vi "JSON to LVJSON.vi"(8 "error in (no error)":errorcluster, 11 "JSON in":string) -> (0 "error out":errorcluster, 3 "Root Element out":T1)   [LabVIEW 2019, in "labview_json.lvlib"]
uses:
  labview_json.lvlib
  Element.ctl
  Element Type.ctl
  <vilib>/Utility/error.llb/Error Cluster From Error Code.vi
  <vilib>/ErrorRing/Error Ring.xnode
  <vilib>/regexp/Match Regular Expression.xnode
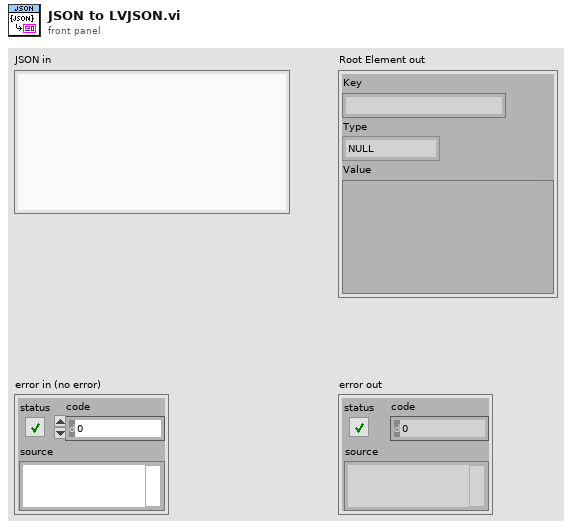
[diagram p1: front panel]
types:
  T1 = typedef "labview_json.lvlib/Element.ctl" = cluster{"Key":string, "Type":T2, "Value":variant}
  T2 = typedef "labview_json.lvlib/Element Type.ctl" = enum8{"NULL", "OBJECT", "ARRAY", "BOOL", "INT", "UINT", "FLOAT", "STRING"}
  T3 = cluster{"Kind":enum8{"Root", "Object", "Array"}, "Name":string, "Values":T1[]}[]
  T4 = cluster{"Kind":enum8{"Root", "Object", "Array"}, "Name":string, "Values":T1[]}
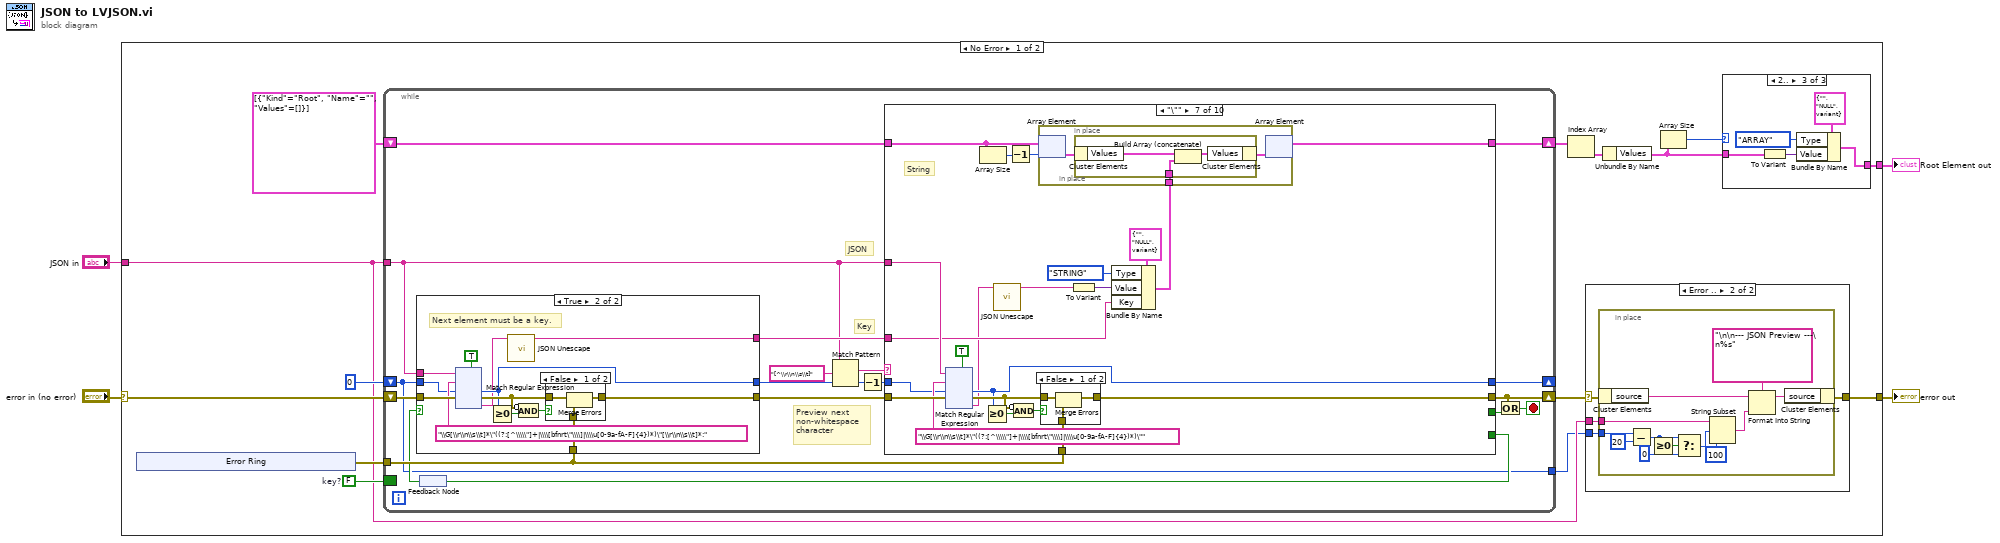
[diagram p0: block diagram]
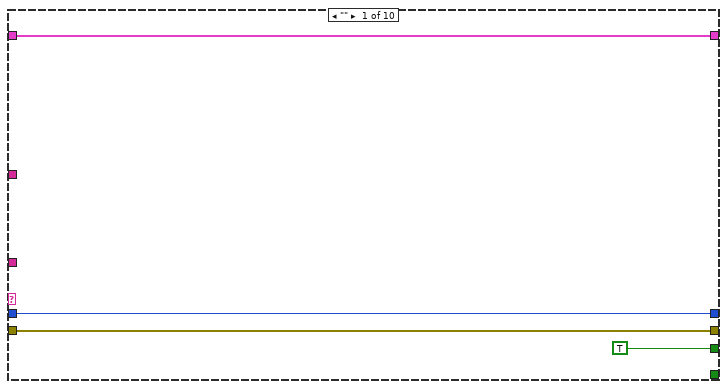
[diagram p5: hidden frame]
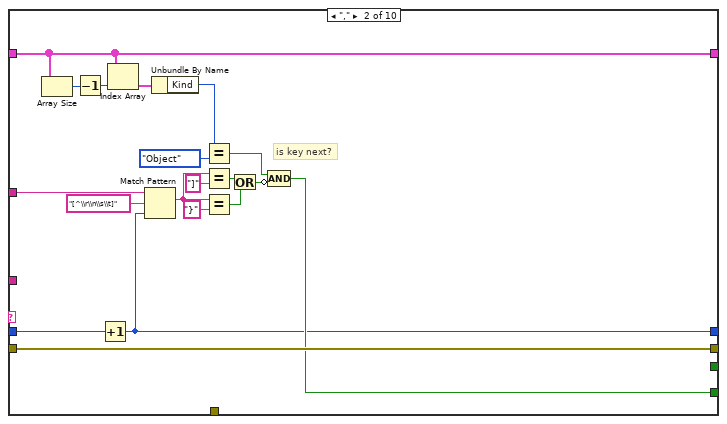
[diagram p6: hidden frame]
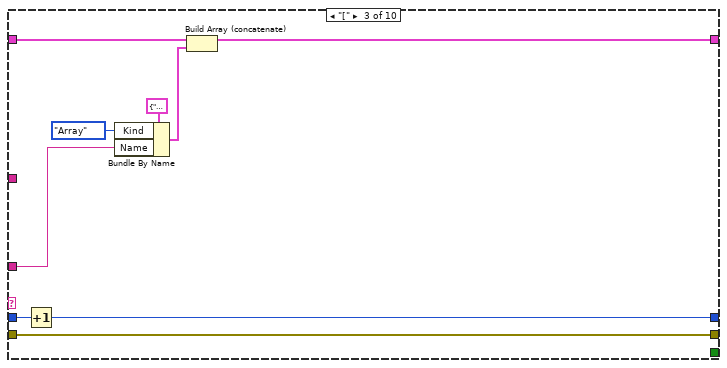
[diagram p7: hidden frame]
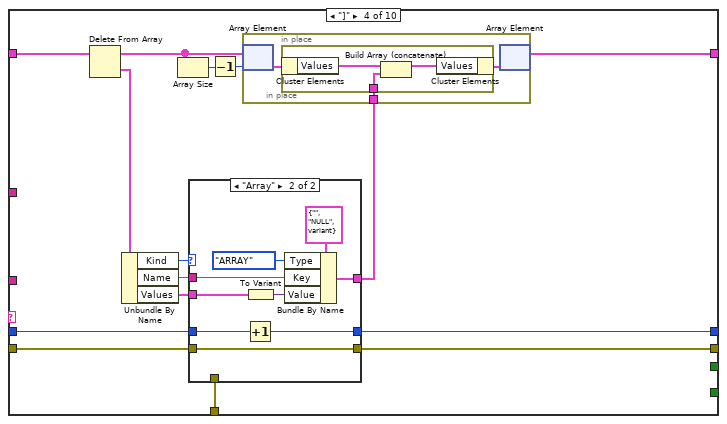
[diagram p8: hidden frame]
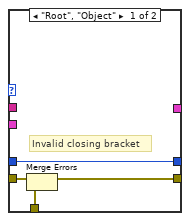
[diagram p9: hidden frame]
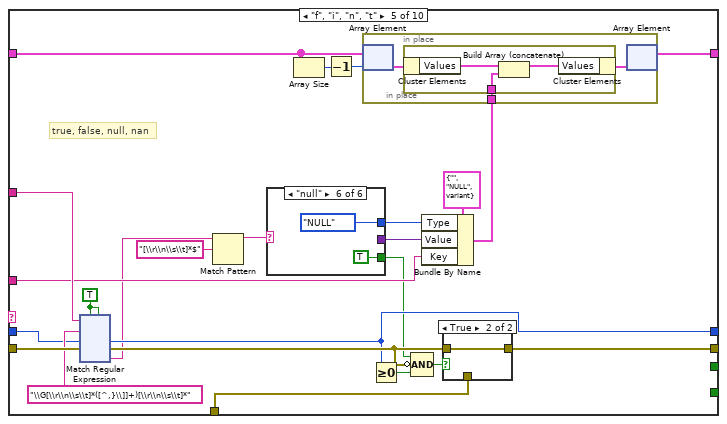
[diagram p10: hidden frame]
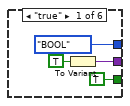
[diagram p11: hidden frame]
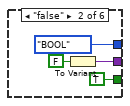
[diagram p12: hidden frame]
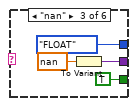
[diagram p13: hidden frame]
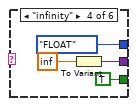
[diagram p14: hidden frame]
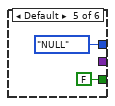
[diagram p15: hidden frame]
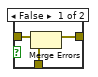
[diagram p16: hidden frame]
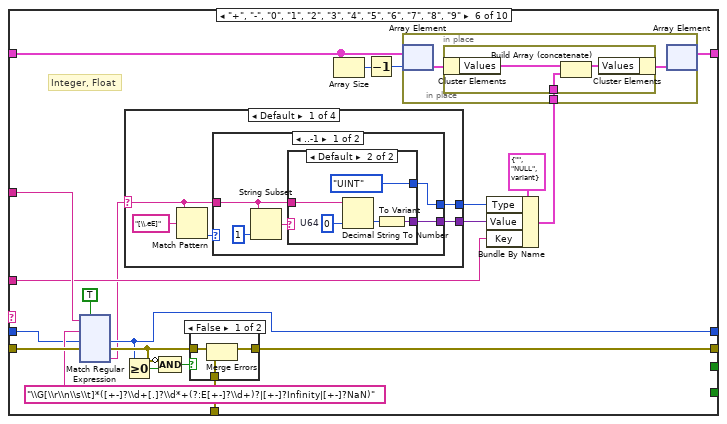
[diagram p17: hidden frame]
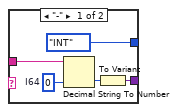
[diagram p18: hidden frame]
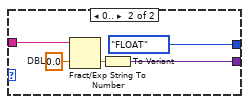
[diagram p19: hidden frame]
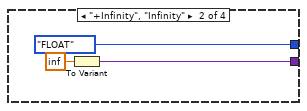
[diagram p20: hidden frame]
diagram:
  n1 = case shown="No Error" "error in (no error)" {
    selector: "error in (no error)" -> [w14 w819]
    tunnel: [w9 _] -> w3
    tunnel: [w8 w819] -> w2
    tunnel: "JSON in" -> [w6 _]
    frame No Error {
      w15 = FALSE  # key?
      n2 = xnode "Error Ring"() -> ("error out"=w13:errorcluster)
      n3 = while {
        tunnel: w6 -> [w48]
        shift-right: [w58] -> w16
        shift-left: T3 [{"Kind"=enum."Root", "Name"="", "Values"=[]}] ("Context") -> [w57]
        shift-right: [w56] -> _
        shift-left: 0 ("Offset in (0)") -> [w40]
        border: w15 -> [_]
        shift-right: [w44] -> w7
        shift-left: w14 -> [w55]
        tunnel: w13 -> [w47]
        tunnel: [w40] -> w5
        stop <- w43 stop-if-true
        # "JSON"
        # "Key"
        # "Preview next\nnon-whitespace\ncharacter"
        n4 = feedback #1() -> (w46:bool)
        n5 = case shown="True" w46 {
          tunnel: w48 -> [_ w72]
          tunnel: w55 -> [w60 w71]
          tunnel: w40 -> [w59 w69]
          tunnel: [w60 w64] -> w51
          tunnel: w47 -> [_ w66]
          tunnel: [w59 w63] -> w53
          tunnel: [_ w61] -> w50
          frame False {
            # "No key"
            # "Next element can be anything"
          }
          frame True {
            # "Next element must be a key."
            n6 = xnode "Match Regular Expression"("input string"=w72, "regular expression"="\\G[\\r\\n\\s\\t]*\"((?:[^\\\\\"]+|\\\\[bfnrt\"\\\\]|\\\\u[0-9a-fA-F]{4})*)\"[\\r\\n\\s\\t]*:", "offset (0)"=w69, "error in"=w71, "multiline? (F)"=TRUE) -> ("offset past match"=w63:i32, "error out"=w65:errorcluster, "submatch 1"=w62:string)  [unwired: 1 in, 3 out]
            n7 = Greater Or Equal To 0?(x=w63) -> (x >= 0?=w68:bool)
            n8 = call "JSON Unescape.vi"("Escaped String"=w62) -> ("String out"=w61:string)  [unwired: 9 in, 1 out]
            n9 = Compound Arithmetic op=AND(invert w65, w68) -> (w67:bool)
            n10 = case shown="False" w67 {
              tunnel: w66 -> [w74 _]
              tunnel: w65 -> [w76 w77]
              tunnel: [w75 w77] -> w64
              frame False {
                n11 = Merge Errors(w76, w74) -> (w75:errorcluster)
              }
              frame True {
              }
            }
          }
        }
        n12 = Match Pattern(string=w48, regular expression="[^\\r\\n\\s\\t]", offset (0)=w53) -> (match substring=w52:string, offset past match=w49:i32)  [unwired: 2 out]
        n13 = Decrement(x=w49) -> (x-1=w45:i32)
        n14 = case shown="\"\\\"\"" w52 {
          tunnel: [TRUE _ _ _ _ _ _ _ _ _] -> w42
          tunnel: w48 -> [_ w202 _ _ w276 w443 w626 w764 _ _]
          tunnel: w45 -> [w195 w201 w220 w228 w265 w432 w617 w767 w775 w809]
          tunnel: [w196 w216 w224 w235 w281 w448 w630 w771 w782 w811] -> w58
          tunnel: w57 -> [w196 w216 w225 w240 w280 w447 w629 w772 w787 w811]
          tunnel: [w195 w198 w218 w229 w269 w436 w620 w760 w776 w809] -> w56
          tunnel: [w194 w200 w219 w232 w267 w434 w619 w766 w779 w808] -> w44
          tunnel: w51 -> [w194 w200 w219 w231 w277 w444 w627 w766 w778 w810]
          tunnel: w50 -> [_ _ w222 _ w264 w431 w616 w769 _ _]
          tunnel: w47 -> [_ _ _ w230 w270 w437 w621 _ w777 w807]
          tunnel: [_ w199 _ _ _ _ _ w761 _ _] -> w41
          frame "" {
          }
          frame "," {
            # "is key next?"
            n15 = Array Size(array=w216) -> (size(s)=w215:i32)
            n16 = Decrement(x=w215) -> (x-1=w214:i32)
            n17 = Increment(x=w201) -> (x+1=w198:i32)
            n18 = Index Array(array=w216, index=w214) -> (element=w213:T4)
            n19 = Match Pattern(string=w202, regular expression="[^\\r\\n\\s\\t]", offset (0)=w198) -> (match substring=w205:string)  [unwired: 3 out]
            n20 = Unbundle By Name(w213) -> ("Kind"=w204:enum8{"Root", "Object", "Array"})
            n21 = Equal?(x=w204, y=enum8{"Root", "Object", "Array"}."Object") -> (x = y?=w208:bool)
            n22 = Equal?(x=w205, y="]") -> (x = y?=w210:bool)
            n23 = Equal?(x=w205, y="}") -> (x = y?=w209:bool)
            n24 = Or(x=w210, y=w209) -> (x .or. y?=w207:bool)
            n25 = Compound Arithmetic op=AND(w208, invert w207) -> (w199:bool)
          }
          frame "[" {
            n26 = Increment(x=w220) -> (x+1=w218:i32)
            n27 = Bundle By Name(cluster=T4 {"Kind"=enum."Root", "Name"="", "Values"=[]} ("Context"), "Kind"=enum8{"Root", "Object", "Array"}."Array", "Name"=w222) -> (w223:T4)
            n28 = Build Array (concatenate)(w225, w223) -> (w224:T3)
          }
          frame "]" {
            n29 = Delete From Array(array=w240) -> (deleted portion=w239:T4, array with subset deleted=w236:T3)  [unwired: 2 in]
            n30 = Unbundle By Name(w239) -> ("Kind"=w234:enum8{"Root", "Object", "Array"}, "Name"=w227:string, "Values"=w233:T1[])
            n31 = Array Size(array=w236) -> (size(s)=w238:i32)
            n32 = case shown="\"Array\"" w234 {
              tunnel: w233 -> [_ w246]
              tunnel: [w243 w252] -> w232
              tunnel: w231 -> [w244 w252]
              tunnel: w230 -> [w242 _]
              tunnel: [w241 w251] -> w229
              tunnel: w228 -> [w241 w253]
              tunnel: [_ w247] -> w226
              tunnel: w227 -> [_ w245]
              frame "Root", "Object" {
                # "Invalid closing bracket"
                n33 = Merge Errors(w244, w242) -> (w243:errorcluster)
              }
              frame "Array" {
                n34 = Increment(x=w253) -> (x+1=w251:i32)
                n35 = To Variant(anything=w246) -> (Variant=w249:variant)
                n36 = Bundle By Name(cluster=T1 {"Key"="", "Type"=enum."NULL", "Value"=variant} ("Value"), "Type"=Element_Type."ARRAY", "Key"=w245, "Value"=w249) -> (w247:T1)
              }
            }
            n37 = Decrement(x=w238) -> (x-1=w237:i32)
            n38 = in-place {
              in-place-border: w226 -> [w255]
              n39 = in-place-array #2(w236, w237) -> (w256:T4)
              n40 = in-place {
                in-place-border: w255 -> [w257]
                n41 = in-place-cluster #3(w256) -> ("Values"=w259:T1[])
                n42 = Build Array (concatenate)(w259, w257) -> (w258:T1[])
                n43 = in-place-cluster #3("Values"=w258) -> (w254:T4)
              }
              n44 = in-place-array #2(w254) -> (w235:T3)  [unwired: 1 out]
            }
          }
          frame "f", "i", "n", "t" {
            w274 = TRUE ("ignore case? (F)")
            # "true, false, null, nan"
            n45 = xnode "Match Regular Expression"("input string"=w276, "regular expression"="\\G[\\r\\n\\s\\t]*([^,}\\]]+)[\\r\\n\\s\\t]*", "offset (0)"=w265, "error in"=w277, "ignore case? (F)"=w274, "multiline? (F)"=w274) -> ("offset past match"=w269:i32, "error out"=w271:errorcluster, "submatch 1"=w261:string)  [unwired: 3 out]
            n46 = Match Pattern(string=w261, regular expression="[\\r\\n\\s\\t]*$") -> (before substring=w260:string)  [unwired: 1 in, 3 out]
            n47 = case shown="\"null\"" w260 {
              tunnel: [Element_Type."BOOL" ("Type") Element_Type."BOOL" ("Type") Element_Type."FLOAT" ("Type") Element_Type."FLOAT" ("Type") Element_Type."NULL" ("Type") Element_Type."NULL" ("Type")] -> w278
              tunnel: [w285 w289 w294 w298 _ _] -> w268
              tunnel: [TRUE TRUE TRUE TRUE FALSE TRUE] -> w263
              frame "true" {
                n48 = To Variant(anything=TRUE) -> (Variant=w285:variant)
              }
              frame "false" {
                n49 = To Variant(anything=FALSE) -> (Variant=w289:variant)
              }
              frame "nan" {
                n50 = To Variant(anything=nan) -> (Variant=w294:variant)
              }
              frame "infinity" {
                n51 = To Variant(anything=inf) -> (Variant=w298:variant)
              }
              frame Default {
              }
              frame "null" {
              }
            }
            n52 = Array Size(array=w280) -> (size(s)=w283:i32)
            n53 = Decrement(x=w283) -> (x-1=w282:i32)
            n54 = Greater Or Equal To 0?(x=w269) -> (x >= 0?=w272:bool)
            n55 = Compound Arithmetic op=AND(w263, invert w271, w272) -> (w273:bool)
            n56 = Bundle By Name(cluster=T1 {"Key"="", "Type"=enum."NULL", "Value"=variant} ("Value"), "Type"=w278, "Value"=w268, "Key"=w264) -> (w266:T1)
            n57 = in-place {
              in-place-border: w266 -> [w425]
              n58 = in-place-array #4(w280, w282) -> (w426:T4)
              n59 = in-place {
                in-place-border: w425 -> [w427]
                n60 = in-place-cluster #5(w426) -> ("Values"=w429:T1[])
                n61 = Build Array (concatenate)(w429, w427) -> (w428:T1[])
                n62 = in-place-cluster #5("Values"=w428) -> (w424:T4)
              }
              n63 = in-place-array #4(w424) -> (w281:T3)  [unwired: 1 out]
            }
            n64 = case shown="True" w273 {
              tunnel: w270 -> [w304 _]
              tunnel: w271 -> [w306 w307]
              tunnel: [w305 w307] -> w267
              frame False {
                n65 = Merge Errors(w306, w304) -> (w305:errorcluster)
              }
              frame True {
              }
            }
          }
          frame "+", "-", "0", "1", "2", "3", "4", "5", "6", "7", "8", "9" {
            # "Integer, Float"
            n66 = xnode "Match Regular Expression"("input string"=w443, "regular expression"="\\G[\\r\\n\\s\\t]*([+-]?\\d+[.]?\\d*+(?:E[+-]?\\d+)?|[+-]?Infinity|[+-]?NaN)", "offset (0)"=w432, "error in"=w444, "ignore case? (F)"=TRUE) -> ("offset past match"=w436:i32, "error out"=w438:errorcluster, "submatch 1"=w430:string)  [unwired: 1 in, 3 out]
            n67 = Greater Or Equal To 0?(x=w436) -> (x >= 0?=w439:bool)
            n68 = case shown="Default" w430 {
              selector: w430 -> [w453 _ _ _]
              tunnel: [w451 Element_Type."FLOAT" ("Type") Element_Type."FLOAT" ("Type") Element_Type."FLOAT" ("Type")] -> w445
              tunnel: [w452 w477 w480 w483] -> w435
              frame Default {
                n69 = Match Pattern(string=w453, regular expression="[\\.eE]") -> (offset past match=w455:i32)  [unwired: 1 in, 3 out]
                n70 = case shown="..-1" w455 {
                  tunnel: w453 -> [w459 w475]
                  tunnel: [w458 w472] -> w452
                  tunnel: [w456 Element_Type."FLOAT" ("Type")] -> w451
                  frame ..-1 {
                    n71 = String Subset(string=w459, length (rest)=1 ("length (rest)")) -> (substring=w457:string)  [unwired: 1 in]
                    n72 = case shown="Default" w457 {
                      tunnel: w459 -> [w465 w470]
                      tunnel: [w462 w467] -> w458
                      tunnel: [Element_Type."INT" ("Type") Element_Type."UINT" ("Type")] -> w456
                      frame "-" {
                        w464 = i64 0  # I64
                        n73 = Decimal String To Number(string=w465, default (0L)=w464) -> (number=w463:i64)  [unwired: 1 in, 1 out]
                        n74 = To Variant(anything=w463) -> (Variant=w462:variant)
                      }
                      frame Default {
                        w469 = u64 0  # U64
                        n75 = Decimal String To Number(string=w470, default (0L)=w469) -> (number=w468:u64)  [unwired: 1 in, 1 out]
                        n76 = To Variant(anything=w468) -> (Variant=w467:variant)
                      }
                    }
                  }
                  frame 0.. {
                    w474 = 0.0  # DBL
                    n77 = Fract/Exp String To Number(string=w475, default (0 dbl)=w474) -> (number=w473:dbl)  [unwired: 2 in, 1 out]
                    n78 = To Variant(anything=w473) -> (Variant=w472:variant)
                  }
                }
              }
              frame "+Infinity", "Infinity" {
                n79 = To Variant(anything=inf) -> (Variant=w477:variant)
              }
              frame "-Infinity" {
                n80 = To Variant(anything=-inf) -> (Variant=w480:variant)
              }
              frame "+NaN", "-NaN", "NaN" {
                n81 = To Variant(anything=nan) -> (Variant=w483:variant)
              }
            }
            n82 = Compound Arithmetic op=AND(invert w438, w439) -> (w440:bool)
            n83 = case shown="False" w440 {
              tunnel: w437 -> [w485 _]
              tunnel: w438 -> [w487 w488]
              tunnel: [w486 w488] -> w434
              frame False {
                n84 = Merge Errors(w487, w485) -> (w486:errorcluster)
              }
              frame True {
              }
            }
            n85 = Array Size(array=w447) -> (size(s)=w450:i32)
            n86 = Decrement(x=w450) -> (x-1=w449:i32)
            n87 = Bundle By Name(cluster=T1 {"Key"="", "Type"=enum."NULL", "Value"=variant} ("Value"), "Type"=w445, "Value"=w435, "Key"=w431) -> (w433:T1)
            n88 = in-place {
              in-place-border: w433 -> [w606]
              n89 = in-place-array #6(w447, w449) -> (w607:T4)
              n90 = in-place {
                in-place-border: w606 -> [w608]
                n91 = in-place-cluster #7(w607) -> ("Values"=w610:T1[])
                n92 = Build Array (concatenate)(w610, w608) -> (w609:T1[])
                n93 = in-place-cluster #7("Values"=w609) -> (w605:T4)
              }
              n94 = in-place-array #6(w605) -> (w448:T3)  [unwired: 1 out]
            }
          }
          frame "\"" {
            # "String"
            n95 = xnode "Match Regular Expression"("input string"=w626, "regular expression"="\\G[\\r\\n\\s\\t]*\"((?:[^\\\\\"]+|\\\\[bfnrt\"\\\\]|\\\\u[0-9a-fA-F]{4})*)\"", "offset (0)"=w617, "error in"=w627, "multiline? (F)"=TRUE ("ignore case? (F)")) -> ("offset past match"=w620:i32, "error out"=w622:errorcluster, "submatch 1"=w613:string)  [unwired: 1 in, 3 out]
            n96 = Array Size(array=w629) -> (size(s)=w632:i32)
            n97 = Greater Or Equal To 0?(x=w620) -> (x >= 0?=w623:bool)
            n98 = call "JSON Unescape.vi"("Escaped String"=w613) -> ("String out"=w612:string)  [unwired: 9 in, 1 out]
            n99 = Decrement(x=w632) -> (x-1=w631:i32)
            n100 = Compound Arithmetic op=AND(invert w622, w623) -> (w624:bool)
            n101 = case shown="False" w624 {
              tunnel: w621 -> [w633 _]
              tunnel: w622 -> [w635 w636]
              tunnel: [w634 w636] -> w619
              frame False {
                n102 = Merge Errors(w635, w633) -> (w634:errorcluster)
              }
              frame True {
              }
            }
            n103 = To Variant(anything=w612) -> (Variant=w611:variant)
            n104 = Bundle By Name(cluster=T1 {"Key"="", "Type"=enum."NULL", "Value"=variant} ("Value"), "Type"=Element_Type."STRING", "Value"=w611, "Key"=w616) -> (w618:T1)
            n105 = in-place {
              in-place-border: w618 -> [w754]
              n106 = in-place-array #8(w629, w631) -> (w755:T4)
              n107 = in-place {
                in-place-border: w754 -> [w756]
                n108 = in-place-cluster #9(w755) -> ("Values"=w758:T1[])
                n109 = Build Array (concatenate)(w758, w756) -> (w757:T1[])
                n110 = in-place-cluster #9("Values"=w757) -> (w753:T4)
              }
              n111 = in-place-array #8(w753) -> (w630:T3)  [unwired: 1 out]
            }
          }
          frame "{" {
            # "Is key next?"
            n112 = Increment(x=w767) -> (x+1=w760:i32)
            n113 = Bundle By Name(cluster=T4 {"Kind"=enum."Root", "Name"="", "Values"=[]} ("Context"), "Kind"=enum8{"Root", "Object", "Array"}."Object", "Name"=w769) -> (w770:T4)
            n114 = Match Pattern(string=w764, regular expression="[^\\r\\n\\s\\t]", offset (0)=w760) -> (match substring=w763:string)  [unwired: 3 out]
            n115 = Build Array (concatenate)(w772, w770) -> (w771:T3)
            n116 = Not Equal?(x=w763, y="}") -> (x != y?=w761:bool)
          }
          frame "}" {
            n117 = Delete From Array(array=w787) -> (deleted portion=w786:T4, array with subset deleted=w783:T3)  [unwired: 2 in]
            n118 = Unbundle By Name(w786) -> ("Kind"=w781:enum8{"Root", "Object", "Array"}, "Name"=w774:string, "Values"=w780:T1[])
            n119 = Array Size(array=w783) -> (size(s)=w785:i32)
            n120 = case shown="\"Object\"" w781 {
              tunnel: w780 -> [_ w793]
              tunnel: [w790 w799] -> w779
              tunnel: w778 -> [w791 w799]
              tunnel: w777 -> [w789 _]
              tunnel: [w788 w798] -> w776
              tunnel: w775 -> [w788 w800]
              tunnel: [_ w794] -> w773
              tunnel: w774 -> [_ w792]
              frame "Root", "Array" {
                # "Invalid closing bracket"
                n121 = Merge Errors(w791, w789) -> (w790:errorcluster)
              }
              frame "Object" {
                n122 = Increment(x=w800) -> (x+1=w798:i32)
                n123 = To Variant(anything=w793) -> (Variant=w796:variant)
                n124 = Bundle By Name(cluster=T1 {"Key"="", "Type"=enum."NULL", "Value"=variant} ("Value"), "Type"=Element_Type."OBJECT", "Key"=w792, "Value"=w796) -> (w794:T1)
              }
            }
            n125 = Decrement(x=w785) -> (x-1=w784:i32)
            n126 = in-place {
              in-place-border: w773 -> [w802]
              n127 = in-place-array #10(w783, w784) -> (w803:T4)
              n128 = in-place {
                in-place-border: w802 -> [w804]
                n129 = in-place-cluster #11(w803) -> ("Values"=w806:T1[])
                n130 = Build Array (concatenate)(w806, w804) -> (w805:T1[])
                n131 = in-place-cluster #11("Values"=w805) -> (w801:T4)
              }
              n132 = in-place-array #10(w801) -> (w782:T3)  [unwired: 1 out]
            }
          }
          frame Default {
            # "Invalid value"
            n133 = Merge Errors(w810, w807) -> (w808:errorcluster)
          }
        }
        n134 = feedback-in #1(w41) -> ()
        n135 = Or(x=w44, y=w42) -> (x .or. y?=w43:bool)
      }
      n136 = Index Array(array=w16) -> (element=w11:T4)  [unwired: 1 in]
      n137 = case shown="Error .." w7 {
        selector: w7 -> [w19 w23]
        tunnel: [w19 w20] -> w8
        tunnel: w6 -> [_ w22]
        tunnel: w5 -> [_ w21]
        frame No Error {
        }
        frame Error {
          n138 = in-place {
            in-place-border: w22 -> [w35]
            in-place-border: w21 -> [w24]
            n139 = in-place-cluster #12(w23) -> ("source"=w32:string)
            n140 = Subtract(x=w24, y=20 ("x")) -> (x-y=w28:i32)
            n141 = Greater Or Equal To 0?(x=w28) -> (x >= 0?=w29:bool)
            n142 = Select(t=w28, s=w29, f=0) -> (s? t:f=w26:i32)
            n143 = String Subset(string=w35, offset (0)=w26, length (rest)=100 ("length (rest)")) -> (substring=w25:string)
            n144 = Format Into String(format string="\n\n--- JSON Preview ---\n%s", initial string=w32, w25) -> (resulting string=w31:string)  [unwired: 1 in, 1 out]
            n145 = in-place-cluster #12("source"=w31) -> (w20:errorcluster)
          }
        }
      }
      n146 = Unbundle By Name(w11) -> ("Values"=w10:T1[])
      n147 = Array Size(array=w10) -> (size(s)=w17:i32)
      n148 = case shown="2.." w17 {
        tunnel: w10 -> [_ w813 w815]
        tunnel: [_ w812 w817] -> w9
        frame ..0 {
        }
        frame 1 {
          n149 = Index Array(array=w813) -> (element=w812:T1)  [unwired: 1 in]
        }
        frame 2.. {
          n150 = To Variant(anything=w815) -> (Variant=w814:variant)
          n151 = Bundle By Name(cluster=T1 {"Key"="", "Type"=enum."NULL", "Value"=variant} ("Value"), "Type"=Element_Type."ARRAY", "Value"=w814) -> (w817:T1)
        }
      }
    }
    frame Error {
    }
  }
  "Root Element out" <- w3
  "error out" <- w2
